vi "TDTSyn-Get RS4 Folder.vi"(11 "error in":errorcluster) -> (8 "folder":string, 15 "error out":errorcluster)   [LabVIEW 2020]
panel:
  in  "Synapse URL":string="http://localhost:24414"
  out "sorted array":cluster{"last mod":timestamp, string}[](array[cluster])
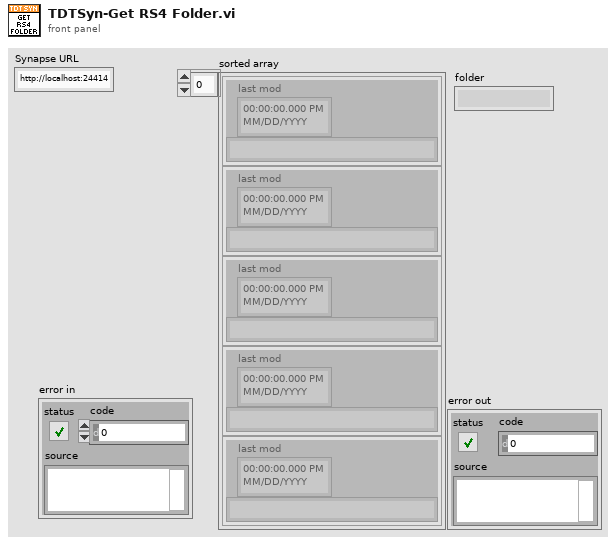
[diagram p1: front panel]
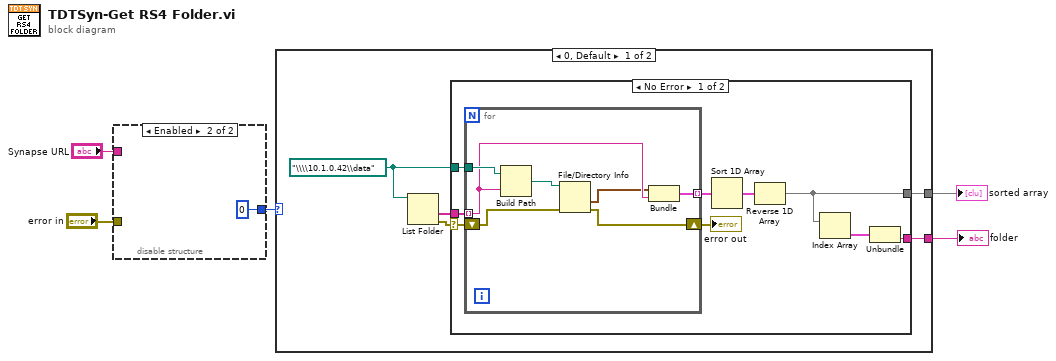
[diagram p0: block diagram]
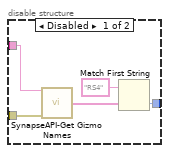
[diagram p2: hidden frame]
diagram:
  n1 = disable-structure shown="Enabled" {
    disable-tunnel: "error in" -> [w10 _]
    disable-tunnel: "Synapse URL" -> [w9 _]
    disable-tunnel: [w6 0 ("index")] -> w1
    frame Disabled {
      n2 = call "SynapseAPI-Get Gizmo Names.vi"("URL"=w9, "error in (no error)"=w10) -> ("names"=w8:string[])  [unwired: 12 in, 1 out]
      n3 = Match First String(2:w8, 3:"RS4" ("string")) -> (0:w6:i32)  [unwired: 1 out]
    }
    frame Enabled {
    }
  }
  n4 = case shown="0, Default" w1 {
    tunnel: [w13 _] -> w5
    tunnel: [w12 _] -> w4
    frame 0, Default {
      w15 = path "\\\\10.1.0.42\\data" ("path")
      n5 = List Folder(path=w15) -> (folder names=w16:string[], error out=w14:errorcluster)  [unwired: 3 in, 2 out]
      n6 = case shown="No Error" w14 {
        selector: w14 -> [w23 _]
        tunnel: w16 -> [w25 _]
        tunnel: w15 -> [w24 _]
        tunnel: [w20 _] -> w13
        tunnel: [w18 _] -> w12
        frame No Error {
          n7 = for {
            tunnel: w25 -> [w28] mode=indexing
            tunnel: w24 -> [w32]
            shift-right: [w29] -> w17
            shift-left: w23 -> [w30]
            tunnel: [w26] -> w22 mode=indexing
            n8 = Build Path(base path=w32, name or relative path=w28) -> (appended path=w31:path)
            n9 = File/Directory Info(path=w31, error in=w30) -> (last mod=w27:timestamp, error out=w29:errorcluster)  [unwired: 5 out]
            n10 = Bundle("last mod"=w27, w28) -> (w26:cluster{"last mod":timestamp, string})  [unwired: 1 in]
          }
          "error out" <- w17
          n11 = Sort 1D Array(array=w22) -> (sorted array=w21:cluster{"last mod":timestamp, string}[])
          n12 = Reverse 1D Array(array=w21) -> (reversed array=w20:cluster{"last mod":timestamp, string}[])
          n13 = Index Array(array=w20) -> (element=w19:cluster{"last mod":timestamp, string})  [unwired: 1 in]
          n14 = Unbundle(w19) -> (w18:string)  [unwired: 1 out]
        }
        frame Error {
        }
      }
    }
    frame -1 {
    }
  }
  "sorted array" <- w5
  "folder" <- w4
